vi "CRYCurve Library Exception Process.vi"(7 "Type In":enum16{"Curves", "Values", "Results", "WFM"}(ring), 8 "Waveform":T1 {"Y dB ref" format="%.1f"; "Y axis" items=["Log", "Lin"]; "Y data" items=["dB", "Lin"]; "X data" items=["dB", "Lin"]}, 9 "Result":T3 {"Margin" format="%.2f"}, 10 "Curve/Value":T5 {"Z data" items=["dB", "Lin"]; "X data" items=["dB", "Lin"]; "Y data" items=["dB", "Lin"]; "Z dB ref" format="%.1f"; "Z axis" items=["Log", "Lin"]; "X dB ref" format="%.1f"; "X axis" items=["Log", "Lin"]; "Y axis" items=["Log", "Lin"]; "Y dB ref" format="%.1f"; "Curve"."z" format="%.2f"; "Curve"."y" format="%.2f"; "Curve"."x" format="%.2f"}, 11 "sAction":string) -> (0 "Waveform Out":T1 {"Y dB ref" format="%.1f"; "Y axis" items=["Log", "Lin"]; "Y data" items=["dB", "Lin"]; "X data" items=["dB", "Lin"]}, 1 "Result Out":T3 {"Margin" format="%.2f"}, 2 "Curve/Value Out":T5 {"Z data" items=["dB", "Lin"]; "X data" items=["dB", "Lin"]; "Y data" items=["dB", "Lin"]; "Z dB ref" format="%.1f"; "Z axis" items=["Log", "Lin"]; "X dB ref" format="%.1f"; "X axis" items=["Log", "Lin"]; "Y axis" items=["Log", "Lin"]; "Y dB ref" format="%.1f"; "Curve"."z" format="%.2f"; "Curve"."y" format="%.2f"; "Curve"."x" format="%.2f"})   [LabVIEW 2013]
uses:
  CRYSystem/Typedef Control/CRYData Cluster Array.ctl
  CRYSystem/Typedef Control/CRYData Cluster.ctl
  CRYSystem/Typedef Control/CRYResult Cluster Array.ctl
  CRYSystem/Typedef Control/CRYResult Cluster.ctl
  CRYSystem/Typedef Control/CRYWaveform Cluster Array.ctl
  CRYSystem/Typedef Control/CRYWaveform Cluster.ctl
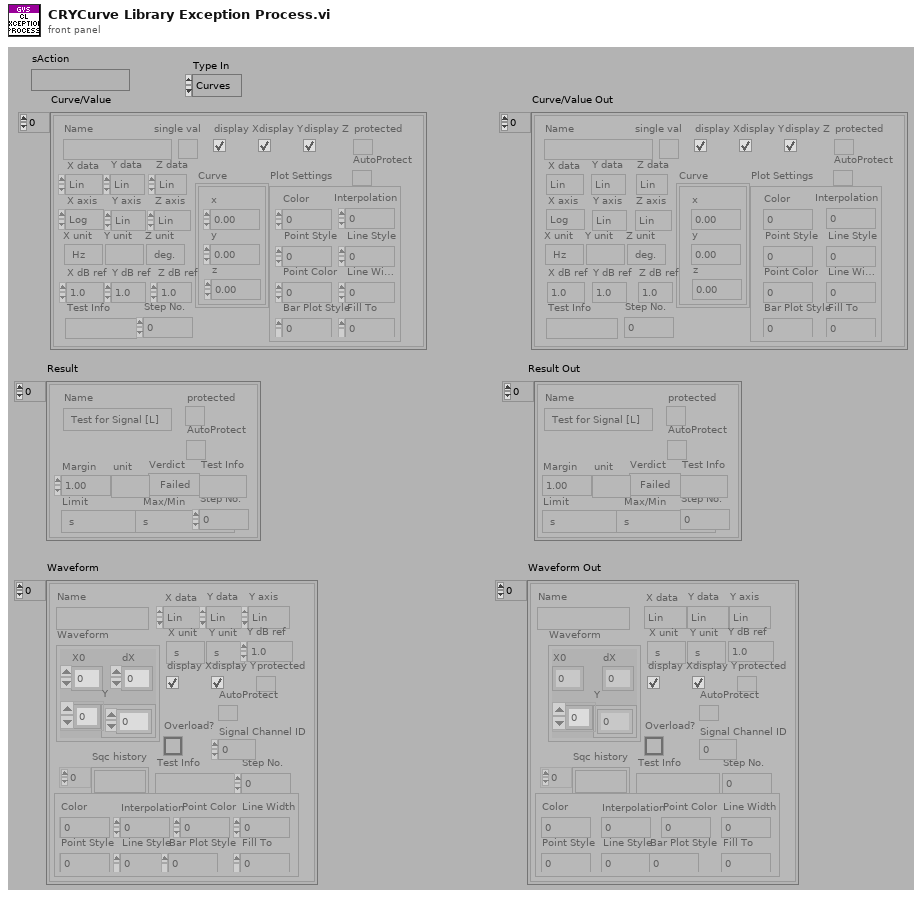
[diagram p1: front panel]
types:
  T1 = typedef "CRYWaveform Cluster Array.ctl" = T2[]
  T2 = typedef "CRYWaveform Cluster.ctl" = cluster{"Waveform":cluster{"X0":dbl, "dX":dbl, "Y":sgl[]}, "X data":u16, "Y data":u16, "Y axis":u16, "X unit":string, "Y unit":string, "Y dB ref":dbl, "display Y":bool, "display X":bool, "Overload?":bool, "Test Info":string, "Step No.":i32, "Name":string, "protected":bool, "Sqc history":string[], "Signal Channel ID":i32, "Plot Settings":cluster{"Color":u32, "Interpolation":u8, "Point Style":u8, "Line Style":u8, "Point Color":u32, "Line Width":u8, "Bar Plot Style":u8, "Fill To":i16}, "AutoProtect":bool}
  T3 = typedef "CRYResult Cluster Array.ctl" = T4[]
  T4 = typedef "CRYResult Cluster.ctl" = cluster{"Name":string, "Margin":dbl, "unit":string, "Verdict":bool, "Limit":string, "Max/Min":string, "protected":bool, "Step No.":i32, "Test Info":string, "AutoProtect":bool}
  T5 = typedef "CRYData Cluster Array.ctl" = T6[]
  T6 = typedef "CRYData Cluster.ctl" = cluster{"Name":string, "Curve":cluster{"x":dbl, "y":dbl, "z":dbl}[], "X data":u16, "Y data":u16, "Z data":u16, "X axis":u16, "Y axis":u16, "Z axis":u16, "X unit":string, "Y unit":string, "Z unit":string, "X dB ref":dbl, "Y dB ref":dbl, "Z dB ref":dbl, "single val":bool, "protected":bool, "display X":bool, "display Y":bool, "display Z":bool, "Test Info":string, "Step No.":i32, "Plot Settings":cluster{"Color":u32, "Interpolation":u8, "Point Style":u8, "Line Style":u8, "Point Color":u32, "Line Width":u8, "Bar Plot Style":u8, "Fill To":i16}, "AutoProtect":bool}
  T7 = enum32{"English", "Chinese", "Korean", "Japanese", "Russian", "Chinese traditional"}
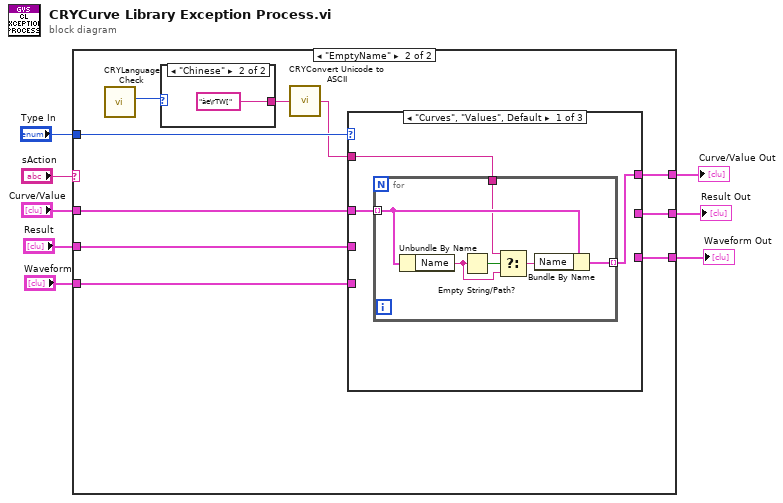
[diagram p0: block diagram]
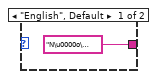
[diagram p3: hidden frame]
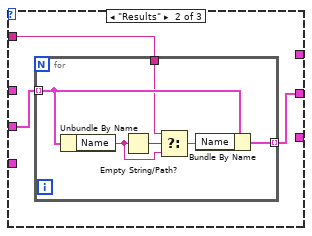
[diagram p4: hidden frame]
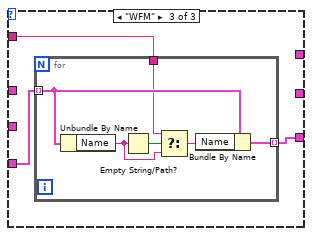
[diagram p5: hidden frame]
diagram:
  n1 = case shown="\"EmptyName\"" "sAction" {
    tunnel: "Type In" -> [_ w21]
    tunnel: "Curve/Value" -> [w11 w20]
    tunnel: "Result" -> [w10 w18]
    tunnel: "Waveform" -> [w9 w16]
    tunnel: [w11 w19] -> w3
    tunnel: [w10 w17] -> w2
    tunnel: [w9 w15] -> w1
    frame Default {
    }
    frame "EmptyName" {
      n2 = call "CRYLanguage Check.vi"() -> ("Language"=w13:T7)  [unwired: 10 in, 1 out]
      n3 = case shown="\"Chinese\"" w13 {
        tunnel: ["N\u0000o\u0000 \u0000N\u0000a\u0000m\u0000e\u0000" "àe\rTW["] -> w14
        frame "English", Default {
        }
        frame "Chinese" {
        }
      }
      n4 = call "CRYConvert Unicode to ASCII.vi"("Unicode"=w14) -> ("ASCII"=w12:string)  [unwired: 4 in]
      n5 = case shown="\"Curves\", \"Values\", Default" w21 {
        tunnel: w20 -> [w26 _ _]
        tunnel: [w25 _ _] -> w19
        tunnel: w18 -> [_ w35 _]
        tunnel: [_ w34 _] -> w17
        tunnel: w16 -> [_ _ w44]
        tunnel: [_ _ w43] -> w15
        tunnel: w12 -> [w24 w33 w42]
        frame "Curves", "Values", Default {
          n6 = for {
            tunnel: w26 -> [w32] mode=indexing
            tunnel: [w31] -> w25 mode=indexing
            tunnel: w24 -> [w27]
            n7 = Unbundle By Name(w32) -> ("Name"=w28:string)
            n8 = Empty String/Path?(string/path=w28) -> (empty?=w30:bool)
            n9 = Select(t=w27, s=w30, f=w28) -> (s? t:f=w29:string)
            n10 = Bundle By Name(cluster=w32, "Name"=w29) -> (w31:T6)
          }
        }
        frame "Results" {
          n11 = for {
            tunnel: w35 -> [w41] mode=indexing
            tunnel: [w40] -> w34 mode=indexing
            tunnel: w33 -> [w36]
            n12 = Unbundle By Name(w41) -> ("Name"=w37:string)
            n13 = Empty String/Path?(string/path=w37) -> (empty?=w39:bool)
            n14 = Select(t=w36, s=w39, f=w37) -> (s? t:f=w38:string)
            n15 = Bundle By Name(cluster=w41, "Name"=w38) -> (w40:T4)
          }
        }
        frame "WFM" {
          n16 = for {
            tunnel: w44 -> [w50] mode=indexing
            tunnel: [w49] -> w43 mode=indexing
            tunnel: w42 -> [w45]
            n17 = Unbundle By Name(w50) -> ("Name"=w46:string)
            n18 = Empty String/Path?(string/path=w46) -> (empty?=w48:bool)
            n19 = Select(t=w45, s=w48, f=w46) -> (s? t:f=w47:string)
            n20 = Bundle By Name(cluster=w50, "Name"=w47) -> (w49:T2)
          }
        }
      }
    }
  }
  "Curve/Value Out" <- w3
  "Waveform Out" <- w1
  "Result Out" <- w2
